vi "OperateDVR.vi"(8 "error in (no error)":errorcluster, 11 "data value reference in":refnum<data-value>) -> (0 "error out":errorcluster, 2 "C":dbl, 3 "data value reference out":refnum<data-value>)   [LabVIEW 2023, in "Arithmetic.lvclass"]
uses:
  Arithmetic.lvclass
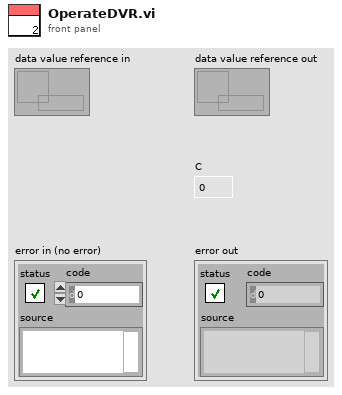
[diagram p1: front panel]
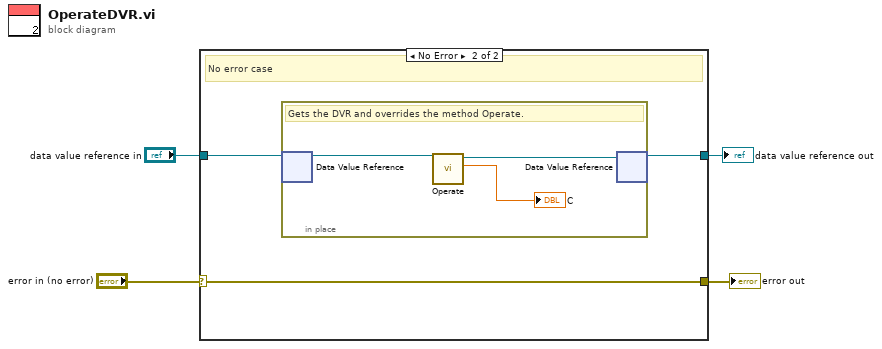
[diagram p0: block diagram]
diagram:
  n1 = case shown="No Error" "error in (no error)" {
    selector: "error in (no error)" -> [w6 w9]
    tunnel: [w6 w9] -> w3
    tunnel: "data value reference in" -> [w5 w8]
    tunnel: [w5 w7] -> w1
    frame Error {
      # "Wire the error cluster across even in the \"No Error\"\ncase so that warnings get propagated."
    }
    frame No Error {
      # "No error case"
      n2 = in-place {
        # "Gets the DVR and overrides the method Operate."
        n3 = in-place-dvr #1(w8) -> (w12:refnum<class "Arithmetic.lvclass">)  [unwired: 1 out]
        n4 = call-dynamic "Operate.vi"("Arithmetic in"=w12) -> ("C"=→"C":dbl, "Arithmetic out"=w11:refnum<class "Arithmetic.lvclass">)  [unwired: 8 in, 1 out]
        n5 = in-place-dvr #1(w11) -> (w7:refnum<data-value>)  [unwired: 1 out]
      }
    }
  }
  "error out" <- w3
  "data value reference out" <- w1
